vi "Get Logging Ref.vi"(8 "error in":errorcluster) -> (0 "error out":errorcluster, 3 "Logger DVR":refnum<data-value>)   [LabVIEW 2016, in "hse-logger.lvlib"]
doc: "Returns the reference (DVR) to the Logger object.\n\n*Warning*\nUse this function only if you are familiar with LVOOP and Data Value References.\n\n____\n(c) HAMPEL SOFTWARE ENGINEERING"
uses:
  hse-logger.lvlib
  Logger/Logger.lvclass
  FGV Actions.ctl
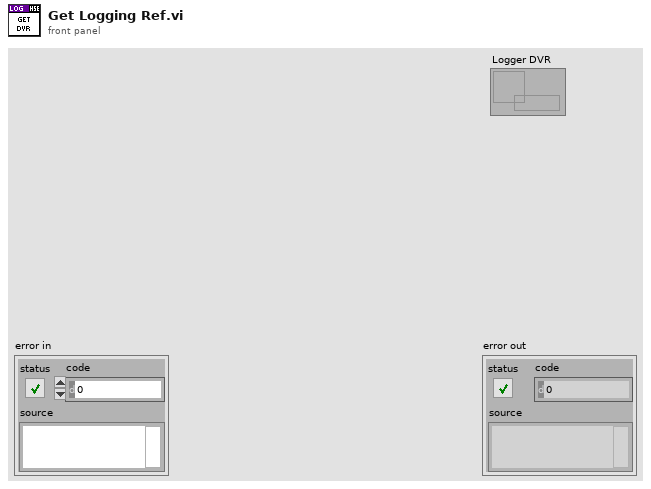
[diagram p1: front panel]
types:
  T1 = typedef "hse-logger.lvlib/FGV Actions.ctl" = enum16{"Set", "Get"}
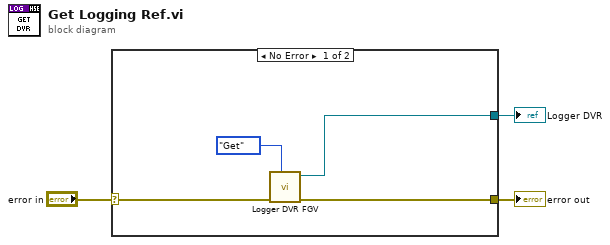
[diagram p0: block diagram]
diagram:
  n1 = case shown="No Error" "error in" {
    selector: "error in" -> [w7 w8]
    tunnel: [w6 w8] -> w2
    tunnel: [w5 _] -> w1
    frame No Error {
      n2 = call "Logger DVR FGV.vi"("FGV Actions"=FGV_Actions."Get", "error in"=w7) -> ("error out"=w6:errorcluster, "Logger DVR"=w5:refnum<data-value>)  [unwired: 8 in]
    }
    frame Error {
    }
  }
  "error out" <- w2
  "Logger DVR" <- w1
